vi "Enable Open Door.vi"(8 "error in (no error)":errorcluster, 10 "Disabled":T1(ring)=enum."Disabled", 11 "Abstract Display Console in":refnum<class "Abstract Display Console.lvclass">) -> (0 "error out":errorcluster, 3 "Abstract Display Console out":refnum<class "Abstract Display Console.lvclass">)   [LabVIEW 2019, in "Abstract Display Console Actor.lvlib" / "Abstract Display Console.lvclass"]
uses:
  Abstract Display Console.lvclass
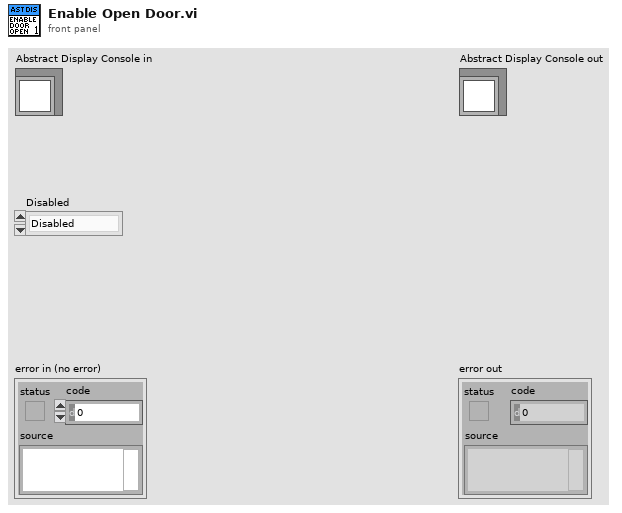
[diagram p1: front panel]
types:
  T1 = enum8{"Enabled", "Disabled", "Disabled and Grayed Out"}
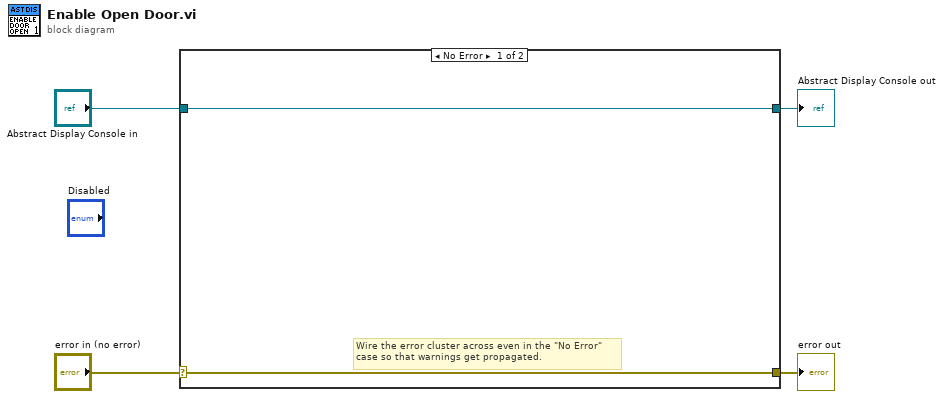
[diagram p0: block diagram]
diagram:
  n1 = case shown="No Error" "error in (no error)" {
    selector: "error in (no error)" -> [w5 w8]
    tunnel: [w5 w8] -> w3
    tunnel: [w6 w7] -> w1
    tunnel: "Abstract Display Console in" -> [w6 w7]
    frame No Error {
      # "Wire the error cluster across even in the \"No Error\"\ncase so that warnings get propagated."
    }
    frame Error {
    }
  }
  "error out" <- w3
  "Abstract Display Console out" <- w1
